vi "Remove Handler.vi"(8 "error in (no error)":errorcluster, 10 "Handler":refnum<class "Handler.lvclass">, 11 "Logger in":refnum<class "Logger.lvclass">) -> (0 "error out":errorcluster, 3 "Logger out":refnum<class "Logger.lvclass">)   [LabVIEW 2017, in "Error Log.lvlib" / "Logger.lvclass"]
doc: "Removes a handler specified by <b>Name</b>. \n\nIf no Handler is found, returns the error \"5030 - Item not found\"."
uses:
  Logger.lvclass
  Handler/Handler.lvclass
  <vilib>/ErrorRing/Error Ring.xnode
  <vilib>/Utility/error.llb/Error Cluster From Error Code.vi
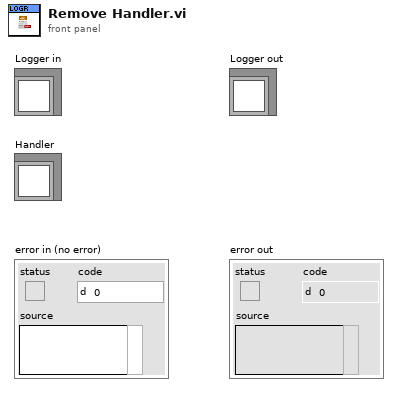
[diagram p1: front panel]
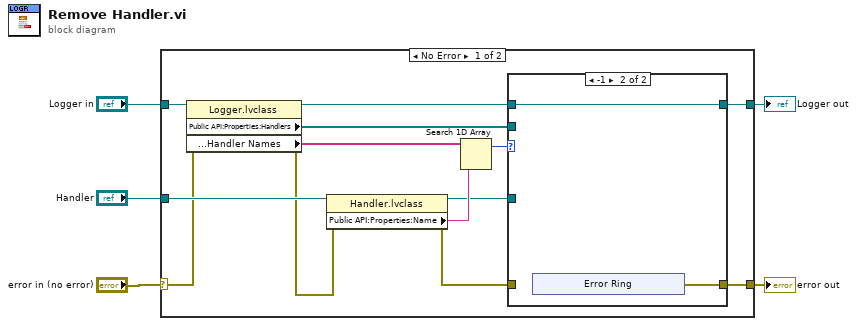
[diagram p0: block diagram]
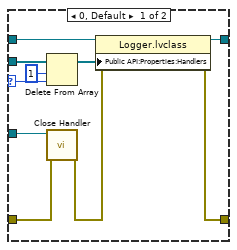
[diagram p2: hidden frame]
diagram:
  n1 = case shown="No Error" "error in (no error)" {
    selector: "error in (no error)" -> [w14 w37]
    tunnel: [w7 w37] -> w4
    tunnel: [w9 w36] -> w2
    tunnel: "Logger in" -> [w17 w36]
    tunnel: "Handler" -> [w18 _]
    frame No Error {
      n2 = property class="Logger.lvclass"(reference=w17, error in=w14) -> (reference out=w10:refnum<class "Logger.lvclass">, error out=w13:errorcluster, "Public API:Properties:Handlers"=w12:refnum<class "Handler.lvclass">[], "Public API:Properties:Handler Names"=w16:string[])
      n3 = property class="Handler.lvclass"(reference=w18, error in=w13) -> (reference out=w6:refnum<class "Handler.lvclass">, error out=w8:errorcluster, "Public API:Properties:Name"=w15:string)
      n4 = Search 1D Array(1D array=w16, element=w15) -> (index of element=w11:i32)  [unwired: 1 in]
      n5 = case shown="-1" w11 {
        selector: w11 -> [w27 _]
        tunnel: w12 -> [w28 _]
        tunnel: w10 -> [w23 w30]
        tunnel: [w22 w30] -> w9
        tunnel: w8 -> [w24 _]
        tunnel: [w19 w29] -> w7
        tunnel: w6 -> [w25 _]
        frame 0, Default {
          n6 = Delete From Array(array=w28, length=1, index=w27) -> (array with subset deleted=w21:refnum<class "Handler.lvclass">[])  [unwired: 1 out]
          n7 = call "Close Handler.vi"("error in (no error)"=w24, "Handler in"=w25) -> ("error out"=w20:errorcluster)  [unwired: 8 in, 1 out]
          n8 = property class="Logger.lvclass"(reference=w23, error in=w20, "Public API:Properties:Handlers"=w21) -> (reference out=w22:refnum<class "Logger.lvclass">, error out=w19:errorcluster)
        }
        frame -1 {
          n9 = xnode "Error Ring"() -> ("error out"=w29:errorcluster)
        }
      }
    }
    frame Error {
    }
  }
  "error out" <- w4
  "Logger out" <- w2
